vi "Drivetrain Targeting.vi"() -> (3 "Drivetrain Center":dbl)   [LabVIEW 2012]
uses:
  Robot Global Data.vi
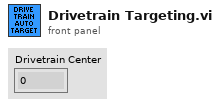
[diagram p1: front panel]
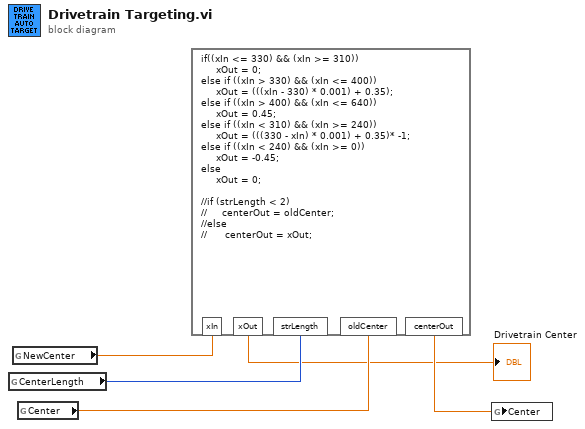
[diagram p0: block diagram]
diagram:
  n1 = global read "Robot Global Data.vi" "CenterLength"() -> (w2:i8)
  n2 = global read "Robot Global Data.vi" "NewCenter"() -> (w3:dbl)
  n3 = global read "Robot Global Data.vi" "Center"() -> (w5:dbl)
  n4 = formula code="if((xIn <= 330) && (xIn >= 310))\n     xOut = 0;\nelse if ((xIn > 330) && (xIn <= 400))\n     xOut = (((xIn - 330) * 0.001) + 0.35);\nelse if ((xIn > 400) && (xIn <= 640))\n     xOut = 0.45;\nelse if ((xIn < 310) && (xIn >= 240))\n     xOut = (((330 - xIn) * 0.001) + 0.35)* -1;\nelse if ((xIn < 240) && (xIn >= 0))\n     xOut = -0.45;\nelse\n     xOut = 0;\n\n//if (strLength < 2) \n//     centerOut = oldCenter;\n//else\n//      centerOut = xOut;"("xIn"=w3, "oldCenter"=w5, "strLength"=w2) -> ("xOut"=→"Drivetrain Center":dbl, "centerOut"=w4:dbl)
  n5 = global write "Robot Global Data.vi" "Center"(w4) -> ()
